vi "Move Tuner per Motor Position.vi"(8 "error in (no error)":errorcluster, 9 "Timeout (60 s)":u8=60, 10 "Positions":cluster{"Motor":u16, "Position":i32}[](array[cluster]) {"Position" min=0; "Motor" items=["Axis 1"=1, "Axis 2"=2, "Axis 3"=3, "Axis 4"=4, "Axis 5"=5, "Axis 6"=6, "Axis 7"=7, "Axis 8"=8]}, 11 "iTuner reference in":refnum<k7>) -> (0 "error out":errorcluster, 2 "Current Positions":cluster{"Motor":u16, "Position":i32}[](array[cluster]) {"Position" min=0; "Motor" items=["Axis 1"=1, "Axis 2"=2, "Axis 3"=3, "Axis 4"=4, "Axis 5"=5, "Axis 6"=6, "Axis 7"=7, "Axis 8"=8]}, 3 "iTuner reference out":refnum<k7>)   [LabVIEW 2016, in "FocusTuner.lvlib"]
doc: "Moves the specified tuner axes to the given positions with timeout."
uses:
  FocusTuner.lvlib
  <instrlib>/Focus iTuner Series/Public/Action-Status/Move Tuner per Motor Position (Motors Array).vi
  <instrlib>/Focus iTuner Series/Public/Data/Query Motor Position (Current Position - All Motors).vi
  <instrlib>/Focus iTuner Series/Focus iTuner Series.lvlib
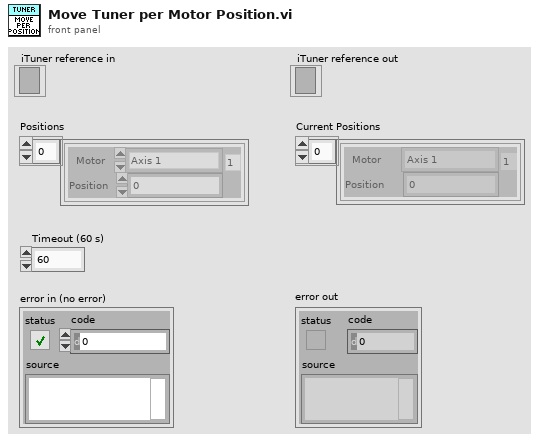
[diagram p1: front panel]
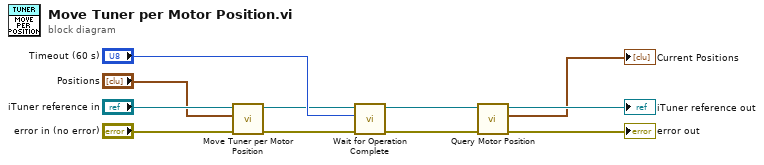
[diagram p0: block diagram]
diagram:
  n1 = call-poly <instrlib>:"Move Tuner per Motor Position.vi"("error in (no error)"="error in (no error)", "Positions"="Positions", "iTuner reference in"="iTuner reference in") -> ("error out"=w4:errorcluster, "iTuner reference out"=w5:refnum<k7>)  [unwired: 7 in]
  n2 = call <instrlib>:"Wait for Operation Complete.vi"("error in (no error)"=w4, "Timeout (60 s)"="Timeout (60 s)", "iTuner reference in"=w5) -> ("error out"=w2:errorcluster, "iTuner reference out"=w3:refnum<k7>)  [unwired: 7 in]
  n3 = call-poly <instrlib>:"Query Motor Position.vi"("error in (no error)"=w2, "iTuner reference in"=w3) -> ("error out"=→"error out":errorcluster, "Positions"=→"Current Positions":cluster{"Motor":u16, "Position":i32}[], "iTuner reference out"=→"iTuner reference out":refnum<k7>)  [unwired: 7 in]
